vi "Console.vi"(6 "Buffer Size":i32=-1, 8 "Last Lines":refnum<vi>, 9 "Remote Console":refnum<vi>, 10 "Queue in":refnum<queue>, 11 "Python":T1) -> ()   [LabVIEW 2022 SP3]
uses:
  PythonCtrl.ctl
  Processors.ctl
panel:
  out "Console":string
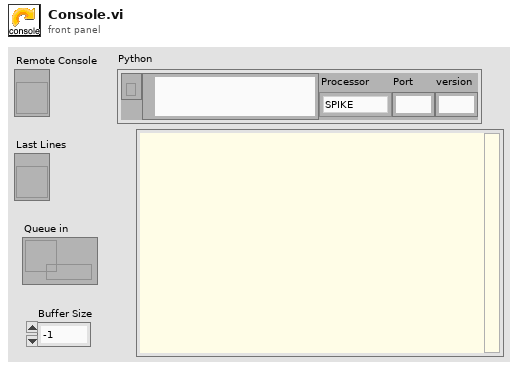
[diagram p1: front panel]
types:
  T1 = typedef "PythonCtrl.ctl" = cluster{"session":refnum<k35>, "PyPath":path, "Processor":T2, "Port":string, "version":string}
  T2 = typedef "Processors.ctl" = enum16{"SPIKE", "Pi", "Pi_ssh", "OpenMV", "Dunio"}
  T3 = enum8{"Enabled", "Disabled", "Disabled and Grayed Out"}
  T4 = typedef "eventvkey.ctl" = enum16{"ASCII", "Enter", "Return", "Shift", "Ctrl", "Alt", "Cmd", "Opt", "Caps", "NumLock", "Clear", "Break", "Up", "Down", "Left", "Right", "Insert", "Delete", "Home", "End", "PageUp", "PageDown", "Escape", "Help", "Pause", "ScrollLock", "F1", "F2", "F3", "F4", "F5", "F6", "F7", "F8", "F9", "F10", "F11", "F12", "F13", "F14", "F15", "F16", "F17", "F18", "F19", "F20", "F21", "F22", "F23", "F24", "Play", "VolumeUp", "VolumeDown", "Mute", "Two Byte Char"}
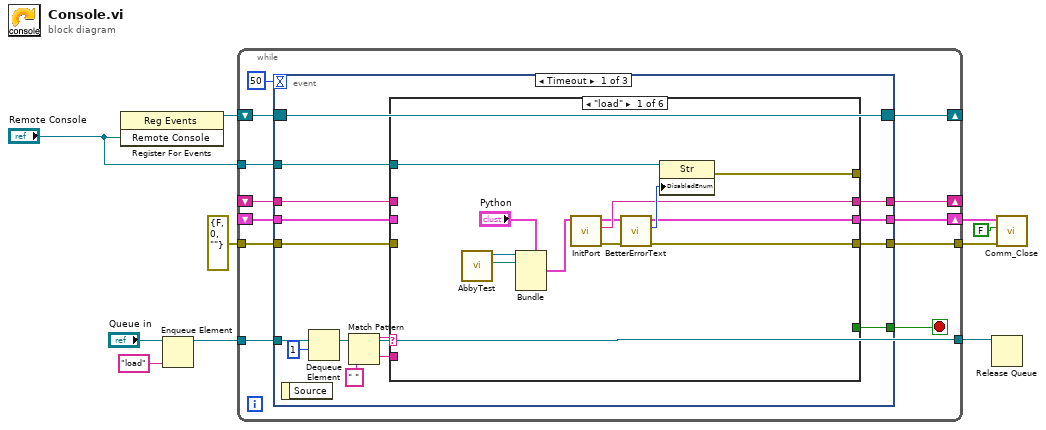
[diagram p0: block diagram]
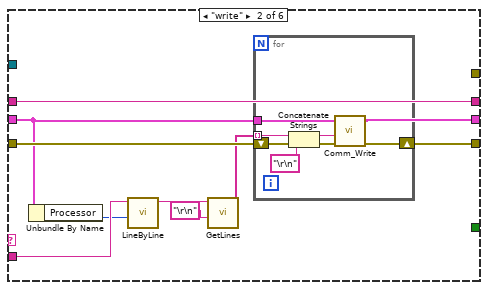
[diagram p2: hidden frame]
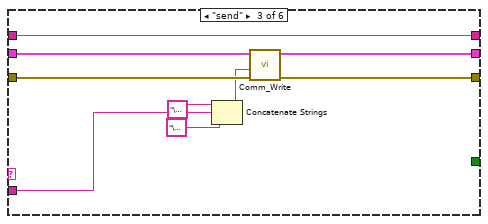
[diagram p3: hidden frame]
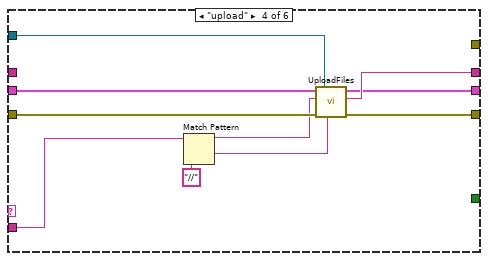
[diagram p4: hidden frame]
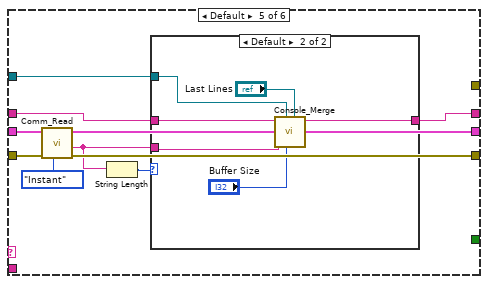
[diagram p5: hidden frame]
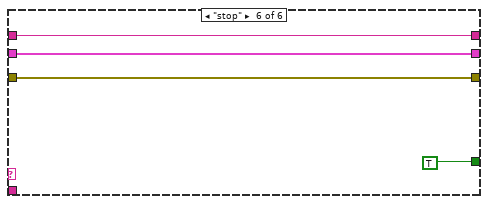
[diagram p7: hidden frame]
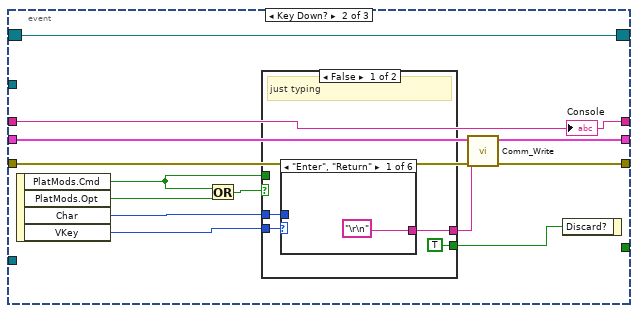
[diagram p8: hidden frame]
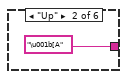
[diagram p9: hidden frame]
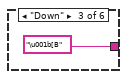
[diagram p10: hidden frame]
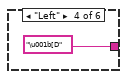
[diagram p11: hidden frame]
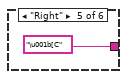
[diagram p12: hidden frame]
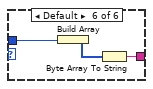
[diagram p13: hidden frame]
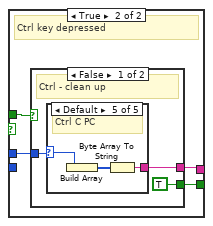
[diagram p14: hidden frame]
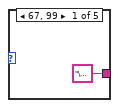
[diagram p15: hidden frame]
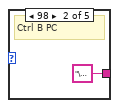
[diagram p16: hidden frame]
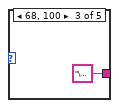
[diagram p17: hidden frame]
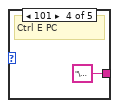
[diagram p18: hidden frame]
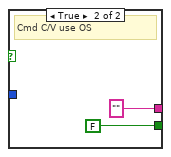
[diagram p19: hidden frame]
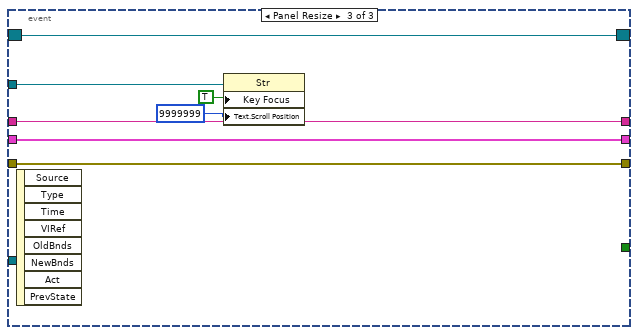
[diagram p20: hidden frame]
diagram:
  n1 = register-events("Remote Console") -> (reference out=w8:refnum<event-registration>)  [unwired: 2 in, 1 out]
  n2 = Enqueue Element(queue="Queue in", element="load") -> (queue out=w4:refnum<queue>)  [unwired: 2 in, 2 out]
  n3 = while {
    shift-right: [w19] -> _
    shift-left: _ -> [w22]
    tunnel: "Remote Console" -> [w17]
    shift-right: [w16] -> _
    shift-left: w8 -> [w18]
    tunnel: w4 -> [w15]
    tunnel: [w15] -> w7
    shift-right: [w14] -> w5
    shift-left: _ -> [w13]
    tunnel: errorcluster {"status"=FALSE, "code"=0, "source"=""} ("error out") -> [w12]
    tunnel: [w11] -> w1
    stop <- w20 stop-if-true
    n4 = event shown="[0] Timeout" {
      selector: w18 -> [w31 w103 w147]
      dyn-events: [w31 w103 w147] -> w16
      timeout: u32 50 ("milliseconds to wait") -> [_ _ _]
      tunnel: w12 -> [w37 w112 w146]
      tunnel: w13 -> [w36 w101 w141]
      tunnel: w22 -> [w35 w104 w145]
      tunnel: [w34 w111 w146] -> w11
      tunnel: [w30 _ _] -> w20
      tunnel: [w33 w104 w145] -> w19
      tunnel: w17 -> [w32 _ w142]
      tunnel: w15 -> [w27 _ _]
      tunnel: [w23 w101 w141] -> w14
      event Timeout {
        n5 = event-data() -> ()  [unwired: 1 in, 1 out]
        n6 = Dequeue Element(queue=w27, timeout in ms (-1)=1) -> (element=w28:string)  [unwired: 1 in, 3 out]
        n7 = Match Pattern(string=w28, regular expression=" ") -> (before substring=w26:string, after substring=w25:string)  [unwired: 1 in, 2 out]
        n8 = case shown="\"load\"" w26 {
          tunnel: w37 -> [_ w55 w69 w79 w89 w99]
          tunnel: w36 -> [_ w48 w63 w76 w81 w97]
          tunnel: w35 -> [_ w56 w70 _ w87 w98]
          tunnel: [w46 w54 w68 w78 w86 w99] -> w34
          tunnel: [w45 w56 w70 w77 w85 w98] -> w33
          tunnel: w32 -> [w44 _ _ w80 w82 _]
          tunnel: [_ _ _ _ _ TRUE] -> w30
          tunnel: w25 -> [_ w53 w65 w74 _ _]
          tunnel: [w43 w48 w63 w71 w81 w97] -> w23
          tunnel: [w42 _ _ _ _ _] -> _
          frame "load" {
            n9 = call "AbbyTest.vi"() -> ("appended path"=w39:path, "Refnum out"=w40:refnum<k35>)  [unwired: 9 in, 1 out]
            n10 = Bundle(cluster="Python", "session"=w40, "PyPath"=w39) -> (w38:T1)  [unwired: 3 in]
            n11 = call "InitPort.vi"("Python"=w38) -> ("error out"=w46:errorcluster, "Console"=w45:string, "Python out"=w43:T1)  [unwired: 8 in]
            n12 = call "BetterErrorText.vi"("error in (no error)"=w46, "Python"=w43) -> ("Disabled"=w47:T3)  [unwired: 8 in, 1 out]
            n13 = property on="Property Node" class="Str"(reference=w44, "DisabledEnum"=w47) -> (error out=w42:errorcluster)  [unwired: 1 in, 1 out]
          }
          frame "write" {
            n14 = Unbundle By Name(w48) -> ("Processor"=w52:T2)
            n15 = call "LineByLine.vi"("Processor"=w52, "Python Code"=w53) -> ("result string"=w51:string)  [unwired: 9 in]
            n16 = call "GetLines.vi"("delimiter"="\r\n", "String"=w51) -> ("Array"=w49:string[])  [unwired: 9 in]
            n17 = for {
              tunnel: w48 -> [w60]
              shift-right: [w61] -> w54
              shift-left: w55 -> [w62]
              tunnel: w49 -> [w59] mode=indexing
              n18 = Concatenate Strings(w59, "\r\n" ("delimiter")) -> (w58:string)
              n19 = call "Comm_Write.vi"("error in (no error)"=w62, "Text to write"=w58, "Python"=w60) -> ("error out"=w61:errorcluster)  [unwired: 7 in, 1 out]
            }
          }
          frame "send" {
            n20 = Concatenate Strings("\u0005" ("queue"), w65, "\u0004" ("queue")) -> (w64:string)
            n21 = call "Comm_Write.vi"("error in (no error)"=w69, "Text to write"=w64, "Python"=w63) -> ("error out"=w68:errorcluster)  [unwired: 7 in, 1 out]
          }
          frame "upload" {
            n22 = Match Pattern(string=w74, regular expression="//") -> (before substring=w73:string, after substring=w72:string)  [unwired: 1 in, 2 out]
            n23 = call "UploadFiles.vi"("Code"=w72, "error in (no error)"=w79, "Python in"=w76, "name"=w73, "Console"=w80) -> ("error out"=w78:errorcluster, "Console out"=w77:string, "Python out"=w71:T1)  [unwired: 4 in]
          }
          frame Default {
            n24 = call "Comm_Read.vi"("Task"=enum16{"Instant", "All", "AllFast", "Params"}."Instant", "error in (no error)"=w89, "Python"=w81) -> ("error out"=w86:errorcluster, "Text read"=w84:string)  [unwired: 7 in]
            n25 = String Length(string=w84) -> (length=w83:i32)
            n26 = case shown="Default" w83 {
              tunnel: w84 -> [_ w93]
              tunnel: w87 -> [w90 w94]
              tunnel: [w90 w96] -> w85
              tunnel: w82 -> [_ w95]
              frame 0 {
              }
              frame Default {
                n27 = call "Console_Merge.vi"("New Lines"="Last Lines", "Buffer Size"="Buffer Size", "Console"=w95, "Text read"=w93, "Console In"=w94) -> ("Console Out"=w96:string)  [unwired: 6 in]
              }
            }
          }
          frame "stop" {
          }
        }
      }
      event Key Down? {
        n28 = event-data() -> ("PlatMods.Cmd"=w105:bool, "PlatMods.Opt"=w108:bool, "Char"=w109:i16, "VKey"=w110:T4)  [unwired: 1 in]
        n29 = Or(x=w105, y=w108) -> (x .or. y?=w107:bool)
        n30 = case shown="False" w107 {
          tunnel: [w116 w127] -> w102
          tunnel: w110 -> [w115 _]
          tunnel: w109 -> [w114 w128]
          tunnel: [TRUE ("Discard?") w126] -> w106
          tunnel: w105 -> [_ w125]
          frame False {
            # "just typing"
            n31 = case shown="\"Enter\", \"Return\"" w115 {
              tunnel: w114 -> [_ _ _ _ _ w124]
              tunnel: ["\r\n" ("replace string (\"\")") "\u001b[A" ("replace string (\"\")") "\u001b[B" ("replace string (\"\")") "\u001b[D" ("replace string (\"\")") "\u001b[C" ("replace string (\"\")") w123] -> w116
              frame "Enter", "Return" {
              }
              frame "Up" {
              }
              frame "Down" {
              }
              frame "Left" {
              }
              frame "Right" {
              }
              frame Default {
                n32 = Build Array(w124) -> (w122:i16[])
                n33 = Byte Array To String(unsigned byte array=w122) -> (string=w123:string)
              }
            }
          }
          frame True {
            # "Ctrl key depressed"
            n34 = case shown="False" w125 {
              tunnel: [w131 "" ("string")] -> w127
              tunnel: w128 -> [w129 _]
              tunnel: [TRUE ("Discard?") FALSE ("Discard?")] -> w126
              frame False {
                # "Ctrl - clean up"
                n35 = case shown="Default" w129 {
                  selector: w129 -> [_ _ _ _ w136]
                  tunnel: ["\u0003" ("string") "\u0002" ("string") "\u0004" ("string") "\u0005" ("string") w137] -> w131
                  frame 67, 99 {
                  }
                  frame 98 {
                    # "Ctrl B PC"
                  }
                  frame 68, 100 {
                  }
                  frame 101 {
                    # "Ctrl E PC"
                  }
                  frame Default {
                    # "Ctrl C PC"
                    n36 = Build Array(w136) -> (w138:i16[])
                    n37 = Byte Array To String(unsigned byte array=w138) -> (string=w137:string)
                  }
                }
              }
              frame True {
                # "Cmd C/V use OS"
              }
            }
          }
        }
        n38 = call "Comm_Write.vi"("error in (no error)"=w112, "Text to write"=w102, "Python"=w101) -> ("error out"=w111:errorcluster)  [unwired: 7 in, 1 out]
        n39 = event-data("Discard?"=w106) -> ()  [unwired: 1 in, 1 out]
        "Console" <- w104
      }
      event Panel Resize {
        n40 = event-data() -> ()  [unwired: 1 in, 8 out]
        n41 = property on="Property Node" class="Str"(reference=w142, "Key Focus"=TRUE, "Text.Scroll Position"=u32 9999999) -> ()  [unwired: 1 in, 2 out]
      }
    }
  }
  n42 = Release Queue(queue=w7) -> ()  [unwired: 2 in, 3 out]
  n43 = call "Comm_Close.vi"("error in (no error)"=w1, "Show Err?"=FALSE, "Python in"=w5) -> ()  [unwired: 7 in, 2 out]
